vi "gds_ber.vi"(8 "error in (no error)":errorcluster, 10 "Recovered Bit Sequence":i8[](array[numeric]), 11 "Received Bit Sequence":i8[](array[numeric]) caption="Key Bit Sequence") -> (0 "error out":errorcluster, 3 "BER":dbl)   [LabVIEW 2012]
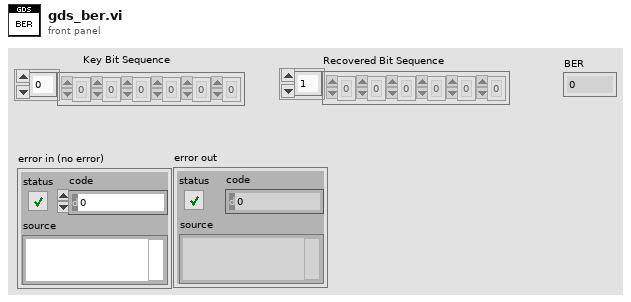
[diagram p1: front panel]
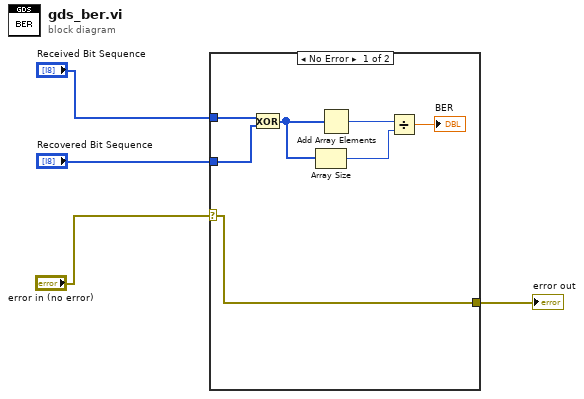
[diagram p0: block diagram]
diagram:
  n1 = case shown="No Error" "error in (no error)" {
    selector: "error in (no error)" -> [w11 w12]
    tunnel: [w11 w12] -> w3
    tunnel: "Received Bit Sequence" -> [w10 _]
    tunnel: "Recovered Bit Sequence" -> [w9 _]
    frame No Error {
      n2 = Exclusive Or(1:w9, 2:w10) -> (0:w8:i8[])
      n3 = Array Size(array=w8) -> (size(s)=w6:i32)
      n4 = Add Array Elements(numeric array=w8) -> (sum=w7:i8)
      n5 = Divide(x=w7, y=w6) -> (x/y=→"BER":dbl)
    }
    frame Error {
    }
  }
  "error out" <- w3
